vi "M06 Solar Cells.vi"(11 "EV3 in":T1) -> ()   [LabVIEW 2016]
uses:
  <vilib>/NXT/Subs/LVHSConnector.ctl
  <vilib>/NXT/LegoClasses/BrickReference/BrickReference.lvclass
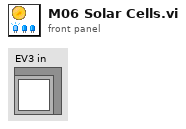
[diagram p1: front panel]
types:
  T1 = typedef "LVHSConnector.ctl" = refnum<class "BrickReference.lvclass">
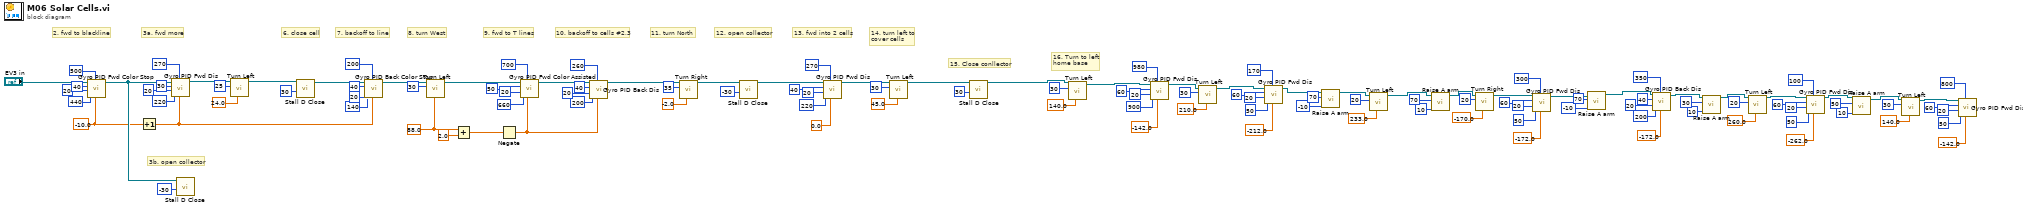
[diagram p0: block diagram]
diagram:
  w109 = sgl 88.0 ("Turning angle")
  w6 = sgl -10.0 ("Target angle")
  # "16. Turn to left \nhome base"
  # "15. Close conllector"
  # "14. turn left to\ncover cells"
  # "13. fwd into 2 cells"
  # "12. open collector"
  # "11. turn North"
  # "10. backoff to cells #2,3"
  # "8. turn West"
  # "7. backoff to line"
  # "9. fwd to T lines"
  # "6. close cell"
  # "3b. open collector"
  # "3a. fwd more"
  # "2. fwd to blackline"
  n1 = call "Gyro PID Fwd Color Stop.vi"("Target angle"=w6, "Threshold to Color"=500, "Threshold to slow"=440, "Min. speed"=20, "Max. speed"=40, "EV3 in"="EV3 in") -> ("EV3 out"=w86:T1)  [unwired: 5 in]
  n2 = Increment(x=w6) -> (x+1=w4:sgl)
  n3 = call "Gyro PID Fwd Dis.vi"("Target angle"=w4, "Threshold to stop"=270, "Threshold to slow"=220, "Min. speed"=20, "Max. speed"=30, "EV3 in"=w86) -> ("EV3 out"=w5:T1)  [unwired: 5 in]
  n4 = call "Stall D Close.vi"("Power"=i8 -30, "NXT/EV3"=w86) -> ()  [unwired: 9 in, 1 out]
  n5 = call "Turn Left.vi"("Turning angle"=sgl 24.0, "Motor B (right)"=i8 25, "EV3 in"=w5) -> ("EV3 out"=w3:T1)  [unwired: 8 in]
  n6 = call "Stall D Close.vi"("Power"=i8 30, "NXT/EV3"=w3) -> ("NXT/EV3"=w104:T1)  [unwired: 9 in]
  n7 = call "Gyro PID Back Color Stop.vi"("Target angle"=w4, "Threshold to Color"=200 ("Threshold to stop"), "Threshold to slow"=140, "Min. speed"=20, "Max. speed"=40, "EV3 in"=w104) -> ("EV3 out"=w85:T1)  [unwired: 5 in]
  n8 = call "Turn Left.vi"("Turning angle"=w109, "Motor B (right)"=i8 30, "EV3 in"=w85) -> ("EV3 out"=w101:T1)  [unwired: 8 in]
  n9 = Add(x=w109, y=sgl 2.0) -> (x+y=w111:sgl)
  n10 = Negate(x=w111) -> (-x=w79:sgl)
  n11 = call "Gyro PID Fwd Color Assisted.vi"("Target angle"=w79, "Threshold to Color"=700 ("Threshold to stop"), "Threshold to slow"=660, "Min. speed"=20, "Max. speed"=50, "EV3 in"=w101) -> ("EV3 out"=w98:T1)  [unwired: 5 in]
  n12 = call "Gyro PID Back Dis.vi"("Target angle"=w79, "Threshold to stop"=260, "Threshold to slow"=200, "Min. speed"=20, "Max. speed"=40, "EV3 in"=w98) -> ("EV3 out"=w84:T1)  [unwired: 5 in]
  n13 = call "Turn Right.vi"("Turning angle"=sgl -2.0, "Motor B (right)"=i8 35, "EV3 in"=w84) -> ("EV3 out"=w96:T1)  [unwired: 8 in]
  n14 = call "Stall D Close.vi"("Power"=i8 -30, "NXT/EV3"=w96) -> ("NXT/EV3"=w91:T1)  [unwired: 9 in]
  n15 = call "Gyro PID Fwd Dis.vi"("Target angle"=sgl 0.0, "Threshold to stop"=270, "Threshold to slow"=220, "Min. speed"=20, "Max. speed"=40, "EV3 in"=w91) -> ("EV3 out"=w89:T1)  [unwired: 5 in]
  n16 = call "Turn Left.vi"("Turning angle"=sgl 45.0, "Motor B (right)"=i8 30, "EV3 in"=w89) -> ("EV3 out"=w77:T1)  [unwired: 8 in]
  n17 = call "Stall D Close.vi"("Power"=i8 30, "NXT/EV3"=w77) -> ("NXT/EV3"=w74:T1)  [unwired: 9 in]
  n18 = call "Turn Left.vi"("Turning angle"=sgl 140.0, "Motor B (right)"=i8 30, "EV3 in"=w74) -> ("EV3 out"=w68:T1)  [unwired: 8 in]
  n19 = call "Gyro PID Fwd Dis.vi"("Target angle"=sgl -142.0, "Threshold to stop"=980, "Threshold to slow"=900, "Min. speed"=20, "Max. speed"=60, "EV3 in"=w68) -> ("EV3 out"=w65:T1)  [unwired: 5 in]
  n20 = call "Turn Left.vi"("Turning angle"=sgl 210.0, "Motor B (right)"=i8 30, "EV3 in"=w65) -> ("EV3 out"=w59:T1)  [unwired: 8 in]
  n21 = call "Gyro PID Fwd Dis.vi"("Target angle"=sgl -212.0, "Threshold to stop"=170, "Threshold to slow"=50, "Min. speed"=20, "Max. speed"=60, "EV3 in"=w59) -> ("EV3 out"=w56:T1)  [unwired: 5 in]
  n22 = call "Raise A arm.vi"("Power"=i8 -10, "Rotation"=70, "EV3 in"=w56) -> ("EV3 out"=w54:T1)  [unwired: 8 in]
  n23 = call "Turn Left.vi"("Turning angle"=sgl 233.0, "Motor B (right)"=i8 20, "EV3 in"=w54) -> ("EV3 out"=w50:T1)  [unwired: 8 in]
  n24 = call "Raise A arm.vi"("Power"=i8 10, "Rotation"=70, "EV3 in"=w50) -> ("EV3 out"=w47:T1)  [unwired: 8 in]
  n25 = call "Turn Right.vi"("Turning angle"=sgl -170.0, "Motor B (right)"=i8 20, "EV3 in"=w47) -> ("EV3 out"=w41:T1)  [unwired: 8 in]
  n26 = call "Gyro PID Fwd Dis.vi"("Target angle"=sgl -172.0, "Threshold to stop"=300, "Threshold to slow"=50, "Min. speed"=20, "Max. speed"=60, "EV3 in"=w41) -> ("EV3 out"=w38:T1)  [unwired: 5 in]
  n27 = call "Raise A arm.vi"("Power"=i8 -10, "Rotation"=70, "EV3 in"=w38) -> ("EV3 out"=w33:T1)  [unwired: 8 in]
  n28 = call "Gyro PID Back Dis.vi"("Target angle"=sgl -172.0, "Threshold to stop"=350, "Threshold to slow"=200, "Min. speed"=20, "Max. speed"=40, "EV3 in"=w33) -> ("EV3 out"=w29:T1)  [unwired: 5 in]
  n29 = call "Raise A arm.vi"("Power"=i8 10, "Rotation"=30, "EV3 in"=w29) -> ("EV3 out"=w26:T1)  [unwired: 8 in]
  n30 = call "Turn Left.vi"("Turning angle"=sgl 260.0, "Motor B (right)"=i8 20, "EV3 in"=w26) -> ("EV3 out"=w20:T1)  [unwired: 8 in]
  n31 = call "Gyro PID Fwd Dis.vi"("Target angle"=sgl -262.0, "Threshold to stop"=100, "Threshold to slow"=50, "Min. speed"=20, "Max. speed"=60, "EV3 in"=w20) -> ("EV3 out"=w17:T1)  [unwired: 5 in]
  n32 = call "Raise A arm.vi"("Power"=i8 10, "Rotation"=50, "EV3 in"=w17) -> ("EV3 out"=w14:T1)  [unwired: 8 in]
  n33 = call "Turn Left.vi"("Turning angle"=sgl 140.0, "Motor B (right)"=i8 30, "EV3 in"=w14) -> ("EV3 out"=w8:T1)  [unwired: 8 in]
  n34 = call "Gyro PID Fwd Dis.vi"("Target angle"=sgl -142.0, "Threshold to stop"=800, "Threshold to slow"=50, "Min. speed"=20, "Max. speed"=60, "EV3 in"=w8) -> ()  [unwired: 5 in, 1 out]
